vi "Get SubPanel Reference.vi"(8 "error in (no error)":errorcluster, 11 "Sound and Vibration in":refnum<class "Sound and Vibration.lvclass">) -> (0 "error out":errorcluster, 2 "VI Ref":refnum<vi>, 3 "Sound and Vibration out":refnum<class "Sound and Vibration.lvclass">)   [LabVIEW 2011, in "Sound and Vibration.lvclass"]
uses:
  Sound and Vibration.lvclass
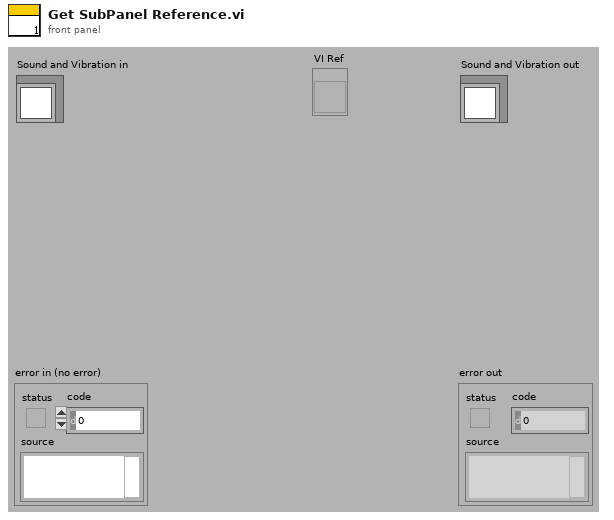
[diagram p1: front panel]
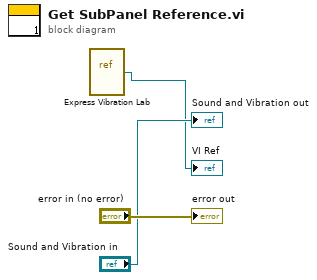
[diagram p0: block diagram]
diagram:
  n1 = vi-ref "Express Vibration Lab.vi"() -> (→"VI Ref":refnum<vi>)
  "error out" <- "error in (no error)"
  "Sound and Vibration out" <- "Sound and Vibration in"
